vi "UPMODE.vi"(4 "error in (no error)":errorcluster, 5 "UPMODE":i32(ring) items=["NORMAL", "ANALOG"], 7 "connection ID":refnum<k5>) -> (0 "error out":errorcluster, 3 "connection ID out":refnum<k5>)   [LabVIEW 2025, in "CAENels FAST-PS.lvlib"]
doc: "The UPMODE command is used to select the update mode of the set-point. There are two possible mode of operation:\n- NORMAL - in this mode of operation the power unit works in the standard update mode. The direct set-point or ramp commands are received using the standard Ethernet communication and they are applied immediately when the command is received. The analog input signal is ignored.\n- ANALOG - in this mode of operation the power unit receives the set-point from its analog input. The analog inputs goes from -10 V up to +10 V. The setting command from the local or remote interface are not accepted. \nNote: this update mode is available only on units that have the analog input. This option has to be communicated at the order of the unit."
uses:
  CAENels FAST-PS.lvlib
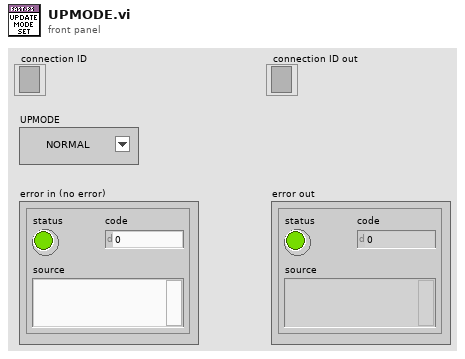
[diagram p1: front panel]
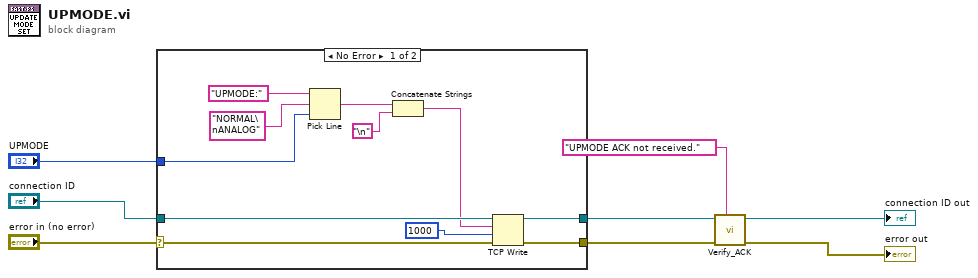
[diagram p0: block diagram]
diagram:
  n1 = case shown="No Error" "error in (no error)" {
    selector: "error in (no error)" -> [w19 w21]
    tunnel: [w18 w21] -> w5
    tunnel: [w17 w20] -> w3
    tunnel: "connection ID" -> [w16 w20]
    tunnel: "UPMODE" -> [w13 _]
    frame No Error {
      n2 = Pick Line(string ("")="UPMODE:", multi-line string="NORMAL\nANALOG" ("string (\"\")"), line index=w13) -> (output string=w12:string)
      n3 = Concatenate Strings(w12, "\n") -> (w10:string)
      n4 = TCP Write(connection ID=w16, data in=w10, error in (no error)=w19, 9:1000 ("timeout ms (25000)")) -> (connection ID out=w17:refnum<k5>, error out=w18:errorcluster)  [unwired: 1 out]
    }
    frame Error {
    }
  }
  n5 = call "Verify_ACK.vi"("error code description"="UPMODE ACK not received.", "error in (no error)"=w5, "connection ID"=w3) -> ("error out"=→"error out":errorcluster, "connection ID out"=→"connection ID out":refnum<k5>)  [unwired: 5 in]
